vi "Pelletron_Status.vi"() -> ()   [LabVIEW 2009, in "AccelNET.lvlib" / "Global_Variables.lvlib"]
uses:
  PelletronStatus.lvclass
  Global_Variables.lvlib
panel:
  in  "AccelNET.lvlib:PelletronStatus.lvclass":refnum<class "PelletronStatus.lvclass">
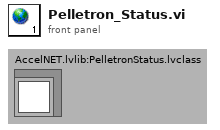
[diagram p1: front panel]
diagram:
